vi "Array Size.vi"() -> ()   [LabVIEW 2017]
panel:
  out "Enum Array Size":i32
  in  "Enum Array":T1(array[ring])
  out "Boolean Array Size":i32
  in  "Boolean Array":bool[](array[boolean])
  out "Array Integer Output":i32
  out "String Array Size":i32
  in  "String Array Input":string[](array[string])
  in  "Numeric Array Input":dbl[](array[numeric])
  out "Array Double Output":dbl
  # "How to use \"Array Size\""
  # "Using then Array Size tool, \nwe can express this value as an integer."
  # "This is an array of four booleans."
  # "Using then Array Size tool, \nwe can express this value as an integer."
  # "Note that this empty value is\nnot expressed in Array Size."
  # "This is an array of three double constants."
  # "Once again, this empty value is\nnot expressed in Array Size."
  # "Using then Array Size tool, \nwe can express this value as an integer."
  # "This is an array of five different\nvalues of the same enum."
  # "This is an array of five strings."
  # "Using then Array Size tool, \nwe can express these values as an integer."
  # "Once again, these empty values are\nnot expressed in Array Size."
  # "Once again, this empty value is\nnot expressed in Array Size."
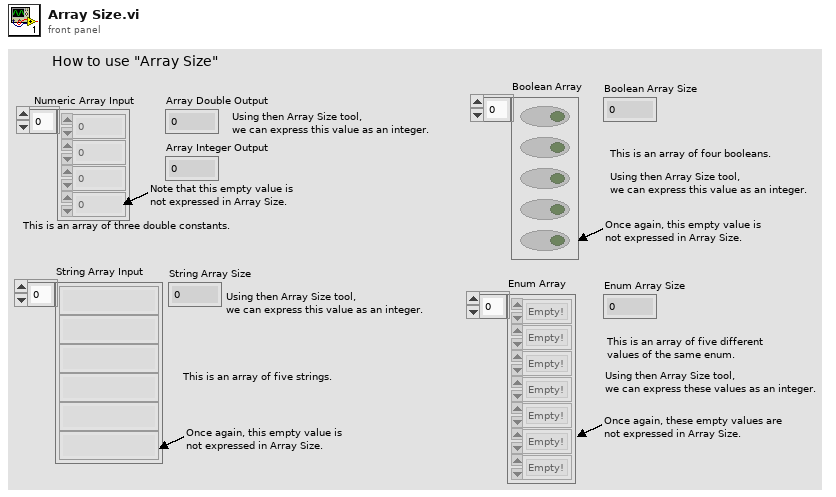
[diagram p1: front panel]
types:
  T1 = enum16{"Empty!", "Also", "Works", "With", "Enums", "It"}[]
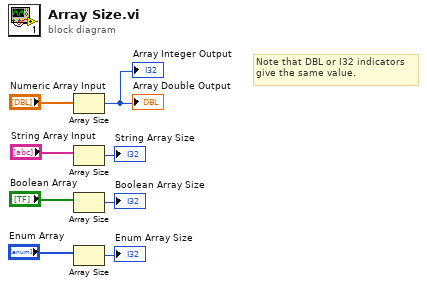
[diagram p0: block diagram]
diagram:
  # "Note that DBL or I32 indicators\ngive the same value."
  n1 = Array Size(array="Numeric Array Input") -> (size(s)=→"Array Double Output" →"Array Integer Output":i32)
  n2 = Array Size(array="String Array Input") -> (size(s)=→"String Array Size":i32)
  n3 = Array Size(array="Boolean Array") -> (size(s)=→"Boolean Array Size":i32)
  n4 = Array Size(array="Enum Array") -> (size(s)=→"Enum Array Size":i32)
